vi "AnalogDemultiplexer_NI5771_3Ghz_Resonance.vi"() -> ()   [LabVIEW 2014]
uses:
  <vilib>/Platform/TimedLoop/XDataNode/timing_clust.ctl
  <vilib>/Platform/TimedLoop/XDataNode/nitl_modes.ctl
  <vilib>/Platform/TimedLoop/XDataNode/wakeup.ctl
  <vilib>/rvi/Emulation/niFpgaGetClockAttributes.vi
  <vilib>/rvi/Emulation/niFpgaSctlEmulationGetInTimedLoop.vi
  <vilib>/rvi/Emulation/niFpgaEmulationReportErrorSimple.vi
  <vilib>/rvi/eio/common/nirviEmuTemplateMethod_errors.vi
  <vilib>/rvi/Emulation/niFpgaCriticalErrorInLSC.vi
  <vilib>/rvi/Emulation/niFpgaEmulationIsFPGAContextNoSignature.vi
  <vilib>/rvi/FIFO/Fifo_Resource/nirvififoEmulationSetSize.vi
  <vilib>/rvi/DataTransferAndStorage/Container/Common/niFpgaContainerGetUniqueNameForEmu.vi
  <vilib>/rvi/FIFO/Fifo_Resource/nirviFifoEmulationQueueMgr.vi
  <instcachedir>/0/nirviFifoEmulationQueueMgr_E5CAEC123FF24DC58D834DCA3CDAA9B5.lvgen/nirviFifoEmulationQueueMgr_E5CAEC123FF24DC58D834DCA3CDAA9B5_002.vi
  <vilib>/rvi/Emulation/niFpgaProcessEmulError.vi
  <vilib>/rvi/errors/niFpgaSetErrorForExecOnDevCompSimple.vi
  <vilib>/rvi/eio/common/nirviEmuReportErrorAndStop.vi
  <vilib>/rvi/FIFO/Fifo_Resource/nirvififoEmulationCreateLock.vi
  <vilib>/rvi/FIFO/Fifo_Resource/nirvififoEmulationObtainLock.vi
  <vilib>/rvi/FIFO/Fifo_Resource/nirvififoEmulationReleaseLock.vi
  <vilib>/rvi/occurrence/nirviWaitOnOccurrenceBase.vi
  <vilib>/rvi/errors/nirviReportUnexpectedCaseInternalError.vi
  <vilib>/rvi/errors/nirviReportUnexpectedCaseInternalError (U32).vi
  <vilib>/rvi/interface/RandomDataEmulation/niFpgaRandomDataHandleErrors.vi
  <vilib>/rvi/FIFO/Fifo_Resource/nirvififoEmulationDetermineInputValidOut.vi
  <vilib>/eio/EIONode/EIONode.xnode
  <vilib>/rvi/DataTransferAndStorage/Container/XNode/niFpgaContainer.xnode
  <vilib>/rvi/FIFO/Fifo_Resource/nirvififoEmulationClear.vi
  <vilib>/Platform/TimedLoop/XDataNode/XDataNode.xnode
  <vilib>/rvi/FIFO/Fifo_Resource/nirvififoEmulationRead.vi
  <vilib>/rvi/interface/RandomDataEmulation/nirviRandomDataFpgaReadWriteTemplate.vi
  <vilib>/rvi/FIFO/Fifo_Resource/nirvififoEmulationWrite.vi
  <vilib>/Platform/TimedLoop/XDataNode/XDNodeRunTimeDep.lvlib
panel:
  in  "CutoffU8 Ch2":u8
  in  "CutoffU8 Ch1":u8
  out "ToHostA2FIFO Overflow":bool
  out "ToHostA1FIFO Overflow":bool
  out "Pixel counter A2":u32
  out "Pixel counter A1":u32
  out "InterloopFIFO Overflow":bool
  in  "BaselineU8 Ch2":u8
  in  "BaselineU8 Ch1":u8
  out "InterloopFIFO timeout":bool
  in  "Clear Interloop FIFO":bool
  out "Acquiring":bool
  in  "Wait for trigger":bool
  in  "Acquire":bool
  in  "Requested pixels A2":u32=100000 caption="Requested pixels"
  in  "Acquire continuously":bool=TRUE
  in  "Requested pixels A1":u32=100000 caption="Requested pixels"
  in  "Samples per pixel":u16=10000 caption="Samples per pixel Acq"
  out "IO Module\\AI Over Range":bool
  in  "User Command Commit":bool
  in  "User Command":u8
  out "User Command Idle":bool
  out "User Command Status":u8
  in  "User Data 0":u16
  in  "User Data 1":u8
  out "PLL Locked":bool
  out "User Error":bool
  out "Configured?":bool
  # "5771 IO module configuration"
  # "Analog demultiplexer V2"
  # "Acquisition control"
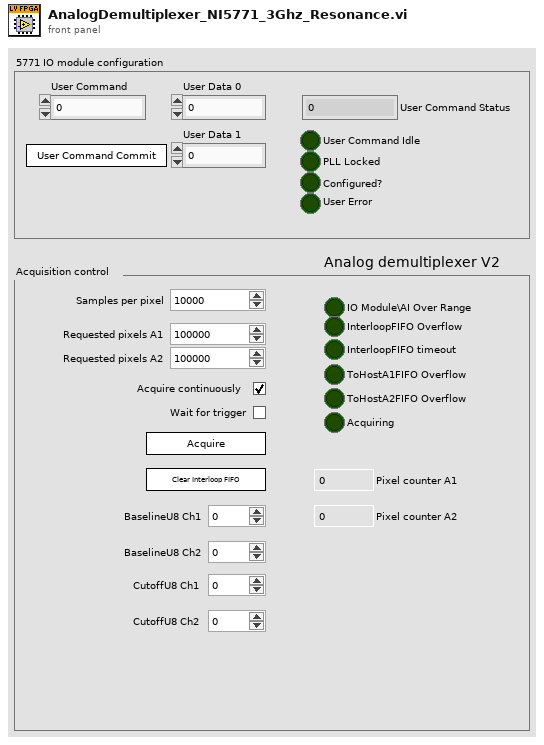
[diagram p1: front panel]
types:
  T1 = typedef "XDNodeRunTimeDep.lvlib/timing_clust.ctl" = cluster{"Expected End [f-1]":u64, "Actual End [f-1]":u64, "Finished Late? [f-1]":bool, "Expected End [i-1]":u64, "Actual End [i-1]":u64, "Finished Late? [i-1]":bool, "Expected Start [i]":u64, "Actual Start [i]":u64, "Expected Start [f]":u64, "Actual Start [f]":u64, "Source Name":string, "Structure Name":string, "Period":i64, "Deadline":i64, "Offset":i64, "Start":i64, "Priority":i32, "Timeout":i32, "Mode":T2, "Wakeup Reason":T3, "Error":errorcluster, "Source Type":string, "Secondary Source Type":string, "Global End Time":u64, "Global Start Time":u64, "Frame Duration":u64, "Iteration Duration":u64, "Assigned CPU":i32, "I/O Scan Engine Mode":u32}
  T2 = typedef "XDNodeRunTimeDep.lvlib/nitl_modes.ctl" = enum32{"No Change", "Process missed periods, maintain original phase", "Discard missed periods, maintain original phase", "Process missed periods, ignore original phase", "Discard missed periods, ignore original phase"}
  T3 = typedef "XDNodeRunTimeDep.lvlib/wakeup.ctl" = enum32{"Normal", "Aborted", "Asynchronous wakeup", "Timing source error", "Timed loop error", "Timeout"}
  T4 = cluster{"IO Module\\AI 1 Data N-7":u8, "IO Module\\AI 1 Data N-6":u8, "IO Module\\AI 1 Data N-5":u8, "IO Module\\AI 1 Data N-4":u8, "IO Module\\AI 1 Data N-3":u8, "IO Module\\AI 1 Data N-2":u8, "IO Module\\AI 1 Data N-1":u8, "IO Module\\AI 1 Data N":u8, "IO Module\\Synchronous Trigger Input":u8}
  T5 = cluster{"IO Module\\AI 0 Data N-7":u8, "IO Module\\AI 0 Data N-6":u8, "IO Module\\AI 0 Data N-5":u8, "IO Module\\AI 0 Data N-4":u8, "IO Module\\AI 0 Data N-3":u8, "IO Module\\AI 0 Data N-2":u8, "IO Module\\AI 0 Data N-1":u8, "IO Module\\AI 0 Data N":u8, "IO Module\\Synchronous Trigger Input":u8}
  T6 = cluster{u16, u16, u16, u16, u16, u16, u16, u16, "IO Module\\Synchronous Trigger Input":u8}
  T7 = cluster{"Output":u32, "Output":u32, "Output":u32, "Output":u32}
  T8 = cluster{"A1 Ch1":u32, "A1 Ch2":u32, "A2 Ch1":u32, "A2 Ch2":u32}
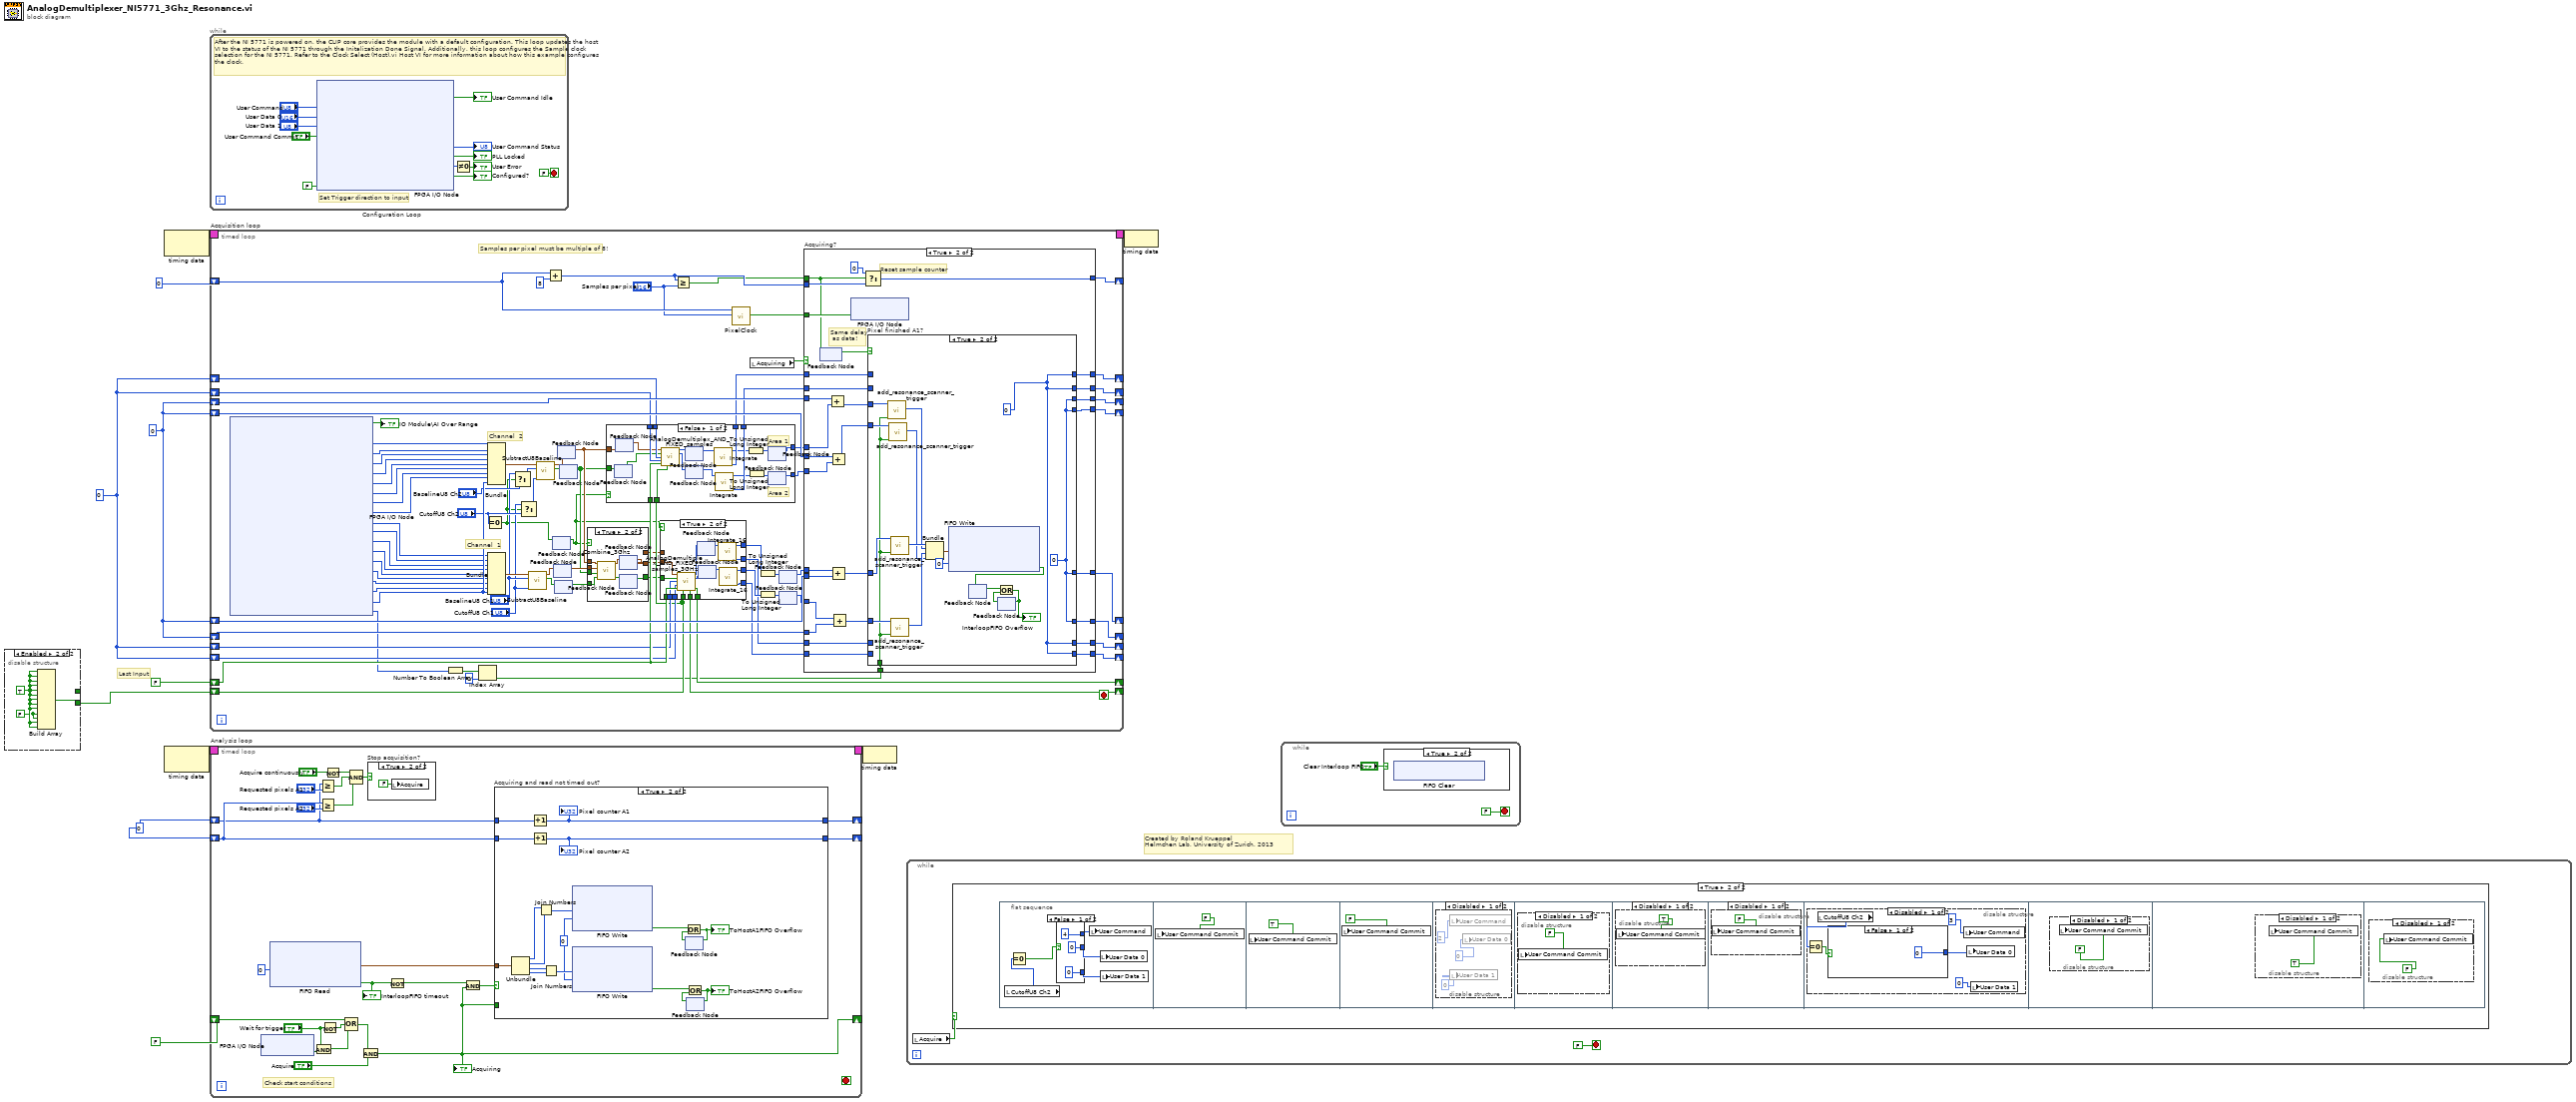
[diagram p0: block diagram]
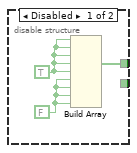
[diagram p2: hidden frame]
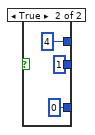
[diagram p4: hidden frame]
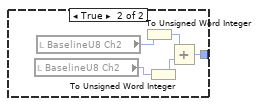
[diagram p9: hidden frame]
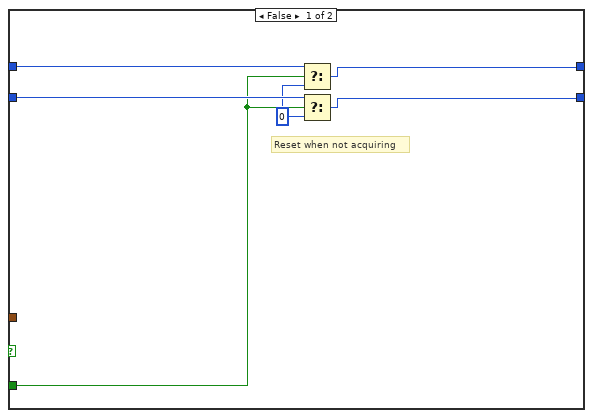
[diagram p15: hidden frame]
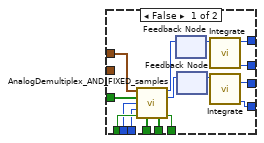
[diagram p17: hidden frame]
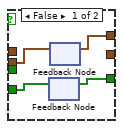
[diagram p18: hidden frame]
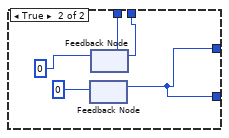
[diagram p19: hidden frame]
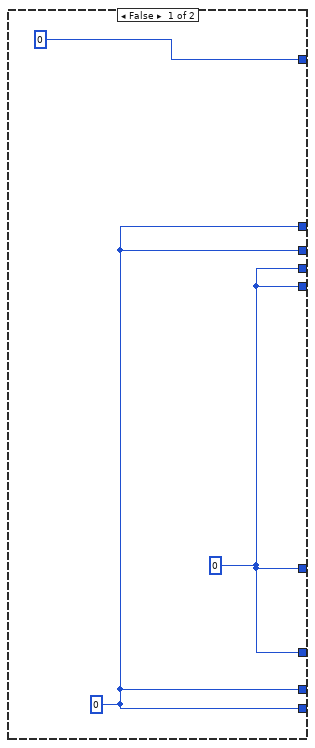
[diagram p20: hidden frame]
diagram:
  w2 = u8 0
  w4 = u32 0
  w6 = u32 0 ("Integrator out")
  # "Last Input"
  # "Created by Roland Krueppel\nHelmchen Lab, University of Zurich, 2013"
  n1 = disable-structure shown="Enabled" {
    disable-tunnel: [w14 _] -> _
    disable-tunnel: [_ w15] -> w1
    frame Disabled {
      w12 = FALSE
      w13 = TRUE
      n2 = Build Array(w13, w13, w13, w13, w13, w12, w12, w12, w12) -> (w14:bool[])
    }
    frame Enabled {
      w16 = FALSE
      w17 = TRUE
      n3 = Build Array(w17, w17, w17, w17, w17, w17, w17, w17, w17, w16, w16, w17, w17) -> (w15:bool[])
    }
  }
  n4 = node-c288() -> (w11:T1)  [unwired: 1 in]
  n5 = node-c288() -> (w9:T1)  [unwired: 1 in]
  n6 = while "Configuration Loop" {
    stop <- FALSE stop-if-true
    # "Set Trigger direction to input"
    # "After the NI 5771 is powered on, the CLIP core provides the module with a default configuration. This loop updates the host VI to the status of the NI 5771 through the Initalization Done Signal. Additionally, this loop configures the Sample clock selection for the NI 5771. Refer to the Clock Select (Host).vi Host VI for more information about how this example configures the clock."
    n7 = xnode "FPGA I/O Node"("IO Module\\User Command"="User Command", "IO Module\\User Data 0"="User Data 0", "IO Module\\User Data 1"="User Data 1", "IO Module\\User Command Commit"="User Command Commit", "IO Module\\Trigger WE"=FALSE ("IO Module\\Trigger WE")) -> ("IO Module\\User Command Idle"=→"User Command Idle":bool, "IO Module\\User Command Status"=→"User Command Status":u8, "IO Module\\PLL Locked"=→"PLL Locked":bool, "IO Module\\User Error"=w24:u8, "IO Module\\Initialization Done"=→"Configured?":bool)  [unwired: 10 in, 10 out]
    n8 = Not Equal To 0?(x=w24) -> (x != 0?=→"User Error":bool)
  }
  n9 = timed-loop "Acquisition loop" {
    timing: w11 -> [_]
    timing-out: [_] -> w10
    shift-right: [w112] -> _
    shift-left: u16 0 -> [w107]
    shift-right: [w92] -> _
    shift-left: w4 -> [w101]
    shift-right: [w91] -> _
    shift-left: w4 -> [w100]
    shift-right: [w93] -> _
    shift-left: w4 -> [w102]
    shift-right: [w94] -> _
    shift-left: w4 -> [w103]
    shift-right: [w84] -> _
    shift-left: FALSE -> [w90]
    shift-right: [w87] -> _
    shift-left: w2 -> [w78]
    shift-right: [w86] -> _
    shift-left: w2 -> [w77]
    shift-right: [w89] -> _
    shift-left: w2 -> [w79]
    shift-right: [w88] -> _
    shift-left: w2 -> [w80]
    shift-right: [w76] -> _
    shift-left: w1 -> [w75]
    stop <- _ stop-if-true
    # "Channel  2"
    # "Channel  1"
    # "Samples per pixel must be multiple of 8!"
    n10 = xnode "FPGA I/O Node"() -> ("IO Module\\AI Over Range"=→"IO Module\\AI Over Range":bool, "IO Module\\AI 1 Data N-7"=w71:u8, "IO Module\\AI 1 Data N-6"=w70:u8, "IO Module\\AI 1 Data N-5"=w69:u8, "IO Module\\AI 1 Data N-4"=w68:u8, "IO Module\\AI 1 Data N-3"=w67:u8, "IO Module\\AI 1 Data N-2"=w66:u8, "IO Module\\AI 1 Data N-1"=w65:u8, "IO Module\\AI 1 Data N"=w64:u8, "IO Module\\AI 0 Data N-7"=w62:u8, "IO Module\\AI 0 Data N-6"=w61:u8, "IO Module\\AI 0 Data N-5"=w60:u8, "IO Module\\AI 0 Data N-4"=w59:u8, "IO Module\\AI 0 Data N-3"=w58:u8, "IO Module\\AI 0 Data N-2"=w57:u8, "IO Module\\AI 0 Data N-1"=w56:u8, "IO Module\\AI 0 Data N"=w55:u8, "IO Module\\Synchronous Trigger Input"=w63:u8, "IO Module\\DIO Port 0 Rd Data"=w54:u8)  [unwired: 19 in, 19 out]
    n11 = Number To Boolean Array(number=w54) -> (Boolean array=w53:bool[])
    n12 = Index Array(array=w53, index=0) -> (element=w73:bool)
    n13 = Equal To 0?(x="CutoffU8 Ch2") -> (x = 0?=w39:bool)
    n14 = Bundle("IO Module\\AI 1 Data N-7"=w71, "IO Module\\AI 1 Data N-6"=w70, "IO Module\\AI 1 Data N-5"=w69, "IO Module\\AI 1 Data N-4"=w68, "IO Module\\AI 1 Data N-3"=w67, "IO Module\\AI 1 Data N-2"=w66, "IO Module\\AI 1 Data N-1"=w65, "IO Module\\AI 1 Data N"=w64, "IO Module\\Synchronous Trigger Input"=w63) -> (w51:T4)  [unwired: 1 in]
    n15 = Bundle("IO Module\\AI 0 Data N-7"=w62, "IO Module\\AI 0 Data N-6"=w61, "IO Module\\AI 0 Data N-5"=w60, "IO Module\\AI 0 Data N-4"=w59, "IO Module\\AI 0 Data N-3"=w58, "IO Module\\AI 0 Data N-2"=w57, "IO Module\\AI 0 Data N-1"=w56, "IO Module\\AI 0 Data N"=w55, "IO Module\\Synchronous Trigger Input"=w63) -> (w72:T5)  [unwired: 1 in]
    n16 = Select(t="BaselineU8 Ch1", s=w39, f="BaselineU8 Ch2") -> (s? t:f=w38:u8)
    n17 = Select(t="CutoffU8 Ch1", s=w39, f="CutoffU8 Ch2") -> (s? t:f=w40:u8)
    n18 = call "SubtractU8Baseline.vi"("Cutoff U8"="CutoffU8 Ch1", "Baseline U8"="BaselineU8 Ch1", "Analog data cluster in"=w72) -> ("Over? Array"=w83:bool[], "Analog data cluster out"=w108:T5)  [unwired: 7 in]
    n19 = call "SubtractU8Baseline.vi"("Cutoff U8"=w40, "Baseline U8"=w38, "Analog data cluster in"=w51) -> ("Over? Array"=w47:bool[], "Analog data cluster out"=w48:T5)  [unwired: 7 in]
    n20 = Add(x=w107, y=u16 8) -> (x+y=w110:u16)
    n21 = feedback #1() -> (w35:bool)  [unwired: 1 in]
    n22 = feedback-in #1(w39) -> ()
    n23 = feedback #2() -> (w50:T5)  [unwired: 1 in]
    n24 = feedback-in #2(w108) -> ()
    n25 = feedback #3() -> (w49:bool[])  [unwired: 1 in]
    n26 = feedback-in #3(w83) -> ()
    n27 = feedback #4() -> (w46:T5)  [unwired: 1 in]
    n28 = feedback-in #4(w48) -> ()
    n29 = feedback #5() -> (w45:bool[])  [unwired: 1 in]
    n30 = feedback-in #5(w47) -> ()
    n31 = case shown="True" w35 {
      tunnel: w50 -> [w145 w156]
      tunnel: w49 -> [w148 w155]
      tunnel: [_ w150] -> w37
      tunnel: [w147 w149] -> w36
      tunnel: w45 -> [_ w154]
      tunnel: w46 -> [_ w153]
      tunnel: [w146 _] -> w34
      frame False {
        n32 = feedback #6() -> (w147:bool[])  [unwired: 1 in]
        n33 = feedback-in #6(w148) -> ()
        n34 = feedback #7() -> (w146:T5)  [unwired: 1 in]
        n35 = feedback-in #7(w145) -> ()
      }
      frame True {
        n36 = call "Combine_3Ghz.vi"("Over? Array AI0"=w155, "Over? Array AI1"=w154, "A0 cluster in"=w156, "A1 cluster in"=w153) -> ("Over? Array Out"=w151:bool[], "A0 cluster out"=w152:T6)  [unwired: 6 in]
        n37 = feedback #8() -> (w150:T6)  [unwired: 1 in]
        n38 = feedback-in #8(w152) -> ()
        n39 = feedback #9() -> (w149:bool[])  [unwired: 1 in]
        n40 = feedback-in #9(w151) -> ()
      }
    }
    n41 = case shown="False" w35 {
      tunnel: [w176 w177] -> w98
      tunnel: [w175 w177] -> w97
      tunnel: w90 -> [w174 _]
      tunnel: [w173 w178] -> w82
      tunnel: [w172 w178] -> w81
      tunnel: w80 -> [w171 _]
      tunnel: w79 -> [w170 _]
      tunnel: w75 -> [w169 _]
      tunnel: w46 -> [w157 _]
      tunnel: w45 -> [w160 _]
      frame False {
        # "Area 2"
        # "Area 1"
        n42 = feedback #10() -> (w159:bool[])  [unwired: 1 in]
        n43 = feedback-in #10(w160) -> ()
        n44 = feedback #11() -> (w158:T5)  [unwired: 1 in]
        n45 = feedback-in #11(w157) -> ()
        n46 = call "AnalogDemultiplex_AND_FIXED_samples.vi"("Analog data cluster"=w158, "Over? Array"=w159, "Last Sample A1"=w170, "Last Sample A2"=w171, "Last? Input"=w174, "array in"=w169) -> ("Data A1 out"=w166:u64, "Data A2 out"=w164:u64)  [unwired: 6 in, 2 out]
        n47 = feedback #12() -> (w165:u64)  [unwired: 1 in]
        n48 = feedback-in #12(w166) -> ()
        n49 = feedback #13() -> (w163:u64)  [unwired: 1 in]
        n50 = feedback-in #13(w164) -> ()
        n51 = call "Integrate.vi"("New samples in"=w165) -> ("Next Sample"=w172:u8, "Sum out"=w162:u16)  [unwired: 9 in]
        n52 = call "Integrate.vi"("New samples in"=w163) -> ("Next Sample"=w173:u8, "Sum out"=w161:u16)  [unwired: 9 in]
        n53 = To Unsigned Long Integer(number=w162) -> (unsigned 32bit integer=w168:u32)
        n54 = To Unsigned Long Integer(number=w161) -> (unsigned 32bit integer=w167:u32)
        n55 = feedback #14() -> (w176:u32)  [unwired: 1 in]
        n56 = feedback-in #14(w168) -> ()
        n57 = feedback #15() -> (w175:u32)  [unwired: 1 in]
        n58 = feedback-in #15(w167) -> ()
      }
      frame True {
        n59 = feedback #16() -> (w177:u32)  [unwired: 1 in]
        n60 = feedback-in #16(u32 0) -> ()
        n61 = feedback #17() -> (w178:u8)  [unwired: 1 in]
        n62 = feedback-in #17(u8 0) -> ()
      }
    }
    n63 = case shown="True" w35 {
      tunnel: [w115 w134] -> w33
      tunnel: [w116 w133] -> w32
      tunnel: w90 -> [w128 w139]
      tunnel: [w127 w144] -> w84
      tunnel: w78 -> [w126 w138]
      tunnel: w77 -> [w125 w137]
      tunnel: [w124 w143] -> w76
      tunnel: w75 -> [w123 w142]
      tunnel: w37 -> [_ w141]
      tunnel: w36 -> [w122 w140]
      tunnel: w34 -> [w121 _]
      tunnel: [w114 w130] -> w31
      tunnel: [w113 w129] -> w30
      frame False {
        n64 = call "AnalogDemultiplex_AND_FIXED_samples.vi"("Analog data cluster"=w121, "Over? Array"=w122, "Last Sample A1"=w126, "Last Sample A2"=w125, "Last? Input"=w128, "array in"=w123) -> ("Data A1 out"=w117:u64, "Data A2 out"=w118:u64, "array out"=w124:bool[], "Last? Output"=w127:bool)  [unwired: 6 in]
        n65 = feedback #18() -> (w119:u64)  [unwired: 1 in]
        n66 = feedback-in #18(w117) -> ()
        n67 = feedback #19() -> (w120:u64)  [unwired: 1 in]
        n68 = feedback-in #19(w118) -> ()
        n69 = call "Integrate.vi"("New samples in"=w119) -> ("Next Sample"=w114:u8, "Sum out"=w115:u16)  [unwired: 9 in]
        n70 = call "Integrate.vi"("New samples in"=w120) -> ("Next Sample"=w113:u8, "Sum out"=w116:u16)  [unwired: 9 in]
      }
      frame True {
        n71 = call "AnalogDemultiplex_AND_FIXED_samples_3GHz.vi"("Analog data cluster"=w141, "Over? Array"=w140, "Last Sample A1"=w138, "Last Sample A2"=w137, "Last? Input"=w139, "array in"=w142) -> ("Data A1 out"=w136:u64, "Data A2 out"=w131:u64, "array out"=w143:bool[], "Last? Output"=w144:bool)  [unwired: 6 in]
        n72 = feedback #20() -> (w135:u64)  [unwired: 1 in]
        n73 = feedback-in #20(w136) -> ()
        n74 = feedback #21() -> (w132:u64)  [unwired: 1 in]
        n75 = feedback-in #21(w131) -> ()
        n76 = call "Integrate_16.vi"("New samples in"=w135) -> ("Next Sample"=w130:u8, "Sum out"=w134:u16)  [unwired: 9 in]
        n77 = call "Integrate_16.vi"("New samples in"=w132) -> ("Next Sample"=w129:u8, "Sum out"=w133:u16)  [unwired: 9 in]
      }
    }
    n78 = Greater Or Equal?(x=w110, y="Samples per pixel") -> (x >= y?=w109:bool)
    n79 = call "PixelClock.vi"("Samples per pixel"="Samples per pixel", "Sample counter"=w107) -> ("Pixel clock"=w106:bool)  [unwired: 9 in]
    n80 = local read "Acquiring"() -> (w95:bool)
    n81 = To Unsigned Long Integer(number=w33) -> (unsigned 32bit integer=w105:u32)
    n82 = To Unsigned Long Integer(number=w32) -> (unsigned 32bit integer=w104:u32)
    n83 = feedback #22() -> (w99:u32)  [unwired: 1 in]
    n84 = feedback-in #22(w105) -> ()
    n85 = feedback #23() -> (w96:u32)  [unwired: 1 in]
    n86 = feedback-in #23(w104) -> ()
    n87 = case "Acquiring?" shown="True" w95 {
      tunnel: [u16 0 ("t") w214] -> w112
      tunnel: w110 -> [_ w213]
      tunnel: w109 -> [_ w203]
      tunnel: w106 -> [_ w207]
      tunnel: w103 -> [_ w193]
      tunnel: w102 -> [_ w212]
      tunnel: w101 -> [_ w196]
      tunnel: w100 -> [_ w211]
      tunnel: w99 -> [_ w194]
      tunnel: w98 -> [_ w210]
      tunnel: w97 -> [_ w209]
      tunnel: w96 -> [_ w195]
      tunnel: [w183 w201] -> w94
      tunnel: [w183 w200] -> w93
      tunnel: [w183 w199] -> w92
      tunnel: [w183 w198] -> w91
      tunnel: [w181 w192] -> w89
      tunnel: [w181 w191] -> w88
      tunnel: [w181 w190] -> w87
      tunnel: [w181 w189] -> w86
      tunnel: w81 -> [_ w188]
      tunnel: w82 -> [_ w187]
      tunnel: w30 -> [_ w186]
      tunnel: w31 -> [_ w185]
      tunnel: w73 -> [_ w184]
      frame False {
        w181 = u8 0 ("t")
        w183 = u32 0
      }
      frame True {
        # "Same delay\n as data!"
        # "Reset sample counter"
        n88 = feedback #24() -> (w202:bool)  [unwired: 1 in]
        n89 = feedback-in #24(w203) -> ()
        n90 = Add(x=w212, y=w210) -> (x+y=w205:u32)
        n91 = Add(x=w211, y=w209) -> (x+y=w204:u32)
        n92 = Add(x=w194, y=w193) -> (x+y=w206:u32)
        n93 = Add(x=w195, y=w196) -> (x+y=w197:u32)
        n94 = xnode "FPGA I/O Node"("Pixel clock"=w207) -> ()  [unwired: 1 in, 1 out]
        n95 = Select(t=u16 0, s=w203, f=w213) -> (s? t:f=w214:u16)
        n96 = case "Pixel finished A1?" shown="True" w202 {
          tunnel: w206 -> [w222 w231]
          tunnel: w205 -> [w221 w229]
          tunnel: w197 -> [w220 w233]
          tunnel: w204 -> [w219 w227]
          tunnel: [w222 w234] -> w201
          tunnel: [w221 w234] -> w200
          tunnel: [w220 w234] -> w199
          tunnel: [w219 w234] -> w198
          tunnel: [w218 w223] -> w192
          tunnel: [w217 w223] -> w191
          tunnel: [w215 w223] -> w190
          tunnel: [w216 w223] -> w189
          tunnel: w188 -> [w218 _]
          tunnel: w187 -> [w217 _]
          tunnel: w186 -> [w216 _]
          tunnel: w185 -> [w215 _]
          tunnel: w184 -> [_ w225]
          frame False {
          }
          frame True {
            w223 = u8 0
            w234 = u32 0
            n97 = call "add_resonance_scanner_trigger.vi"("Trigger"=w225, "Input"=w229) -> ("Output"=w228:u32)  [unwired: 9 in]
            n98 = call "add_resonance_scanner_trigger.vi"("Trigger"=w225, "Input"=w227) -> ("Output"=w226:u32)  [unwired: 9 in]
            n99 = call "add_resonance_scanner_trigger.vi"("Trigger"=w225, "Input"=w231) -> ("Output"=w230:u32)  [unwired: 9 in]
            n100 = call "add_resonance_scanner_trigger.vi"("Trigger"=w225, "Input"=w233) -> ("Output"=w232:u32)  [unwired: 9 in]
            n101 = Bundle("Output"=w230, "Output"=w228, "Output"=w232, "Output"=w226) -> (w224:T7)  [unwired: 1 in]
            n102 = xnode ("FIFO Write")("Element"=w224, "Timeout"=0) -> ("Timed Out?"=w235:bool)  [unwired: 1 in, 1 out]
            n103 = feedback #25() -> (w236:bool)  [unwired: 1 in]
            n104 = feedback-in #25(w235) -> ()
            n105 = feedback #26() -> (w237:bool)  [unwired: 1 in]
            n106 = Or(x=w236, y=w237) -> (x .or. y?=w238:bool)
            "InterloopFIFO Overflow" <- w238
            n107 = feedback-in #26(w238) -> ()
          }
        }
      }
    }
  }
  n108 = timed-loop "Analysis loop" {
    timing: w9 -> [_]
    timing-out: [_] -> w8
    shift-right: [w242] -> _
    shift-left: FALSE -> [w252]
    shift-right: [w245] -> _
    shift-left: w6 -> [w246]
    shift-right: [w244] -> _
    shift-left: w6 -> [w247]
    stop <- _ stop-if-true
    # "Check start conditions"
    n109 = xnode "FPGA I/O Node"() -> ("TriggerIn"=w257:bool)  [unwired: 1 in, 1 out]
    n110 = xnode ("FIFO Read")("Timeout"=0) -> ("Element"=w243:T8, "Timed Out?"=w249:bool)  [unwired: 1 in, 1 out]
    "InterloopFIFO timeout" <- w249
    n111 = And(x="Wait for trigger", y=w257) -> (x .and. y?=w254:bool)
    n112 = Greater Or Equal?(x=w246, y="Requested pixels A1") -> (x >= y?=w260:bool)
    n113 = Greater Or Equal?(x=w247, y="Requested pixels A2") -> (x >= y?=w259:bool)
    n114 = Not(x="Wait for trigger") -> (.not. x?=w255:bool)
    n115 = Not(x="Acquire continuously") -> (.not. x?=w261:bool)
    n116 = Compound Arithmetic op=OR(w252, w255, w254) -> (w253:bool)
    n117 = Compound Arithmetic op=AND(w261, w260, w259) -> (w251:bool)
    n118 = And(x=w253, y="Acquire") -> (x .and. y?=w242:bool)
    "Acquiring" <- w242
    n119 = case "Stop acquisition?" shown="True" w251 {
      frame False {
      }
      frame True {
        n120 = local write "Acquire"(FALSE ("Acquire")) -> ()
      }
    }
    n121 = Not(x=w249) -> (.not. x?=w248:bool)
    n122 = And(x=w248, y=w242) -> (x .and. y?=w250:bool)
    n123 = case "Acquiring and read not timed out?" shown="True" w250 {
      tunnel: w247 -> [w269 w288]
      tunnel: w246 -> [w271 w289]
      tunnel: [w270 w286] -> w245
      tunnel: [w268 w287] -> w244
      tunnel: w243 -> [_ w285]
      tunnel: w242 -> [w267 _]
      frame False {
        w266 = u32 0 ("f")
        # "Reset when not acquiring"
        n124 = Select(t=w271, s=w267, f=w266) -> (s? t:f=w270:u32)
        n125 = Select(t=w269, s=w267, f=w266) -> (s? t:f=w268:u32)
      }
      frame True {
        w278 = 0 ("Timeout")
        n126 = Unbundle(w285) -> ("A1 Ch1"=w284:u32, "A1 Ch2"=w283:u32, "A2 Ch1"=w281:u32, "A2 Ch2"=w280:u32)
        n127 = Increment(x=w289) -> (x+1=w286:u32)
        "Pixel counter A1" <- w286
        n128 = Increment(x=w288) -> (x+1=w287:u32)
        "Pixel counter A2" <- w287
        n129 = Join Numbers(hi=w284, lo=w283) -> ((hi.lo)=w282:u64)
        n130 = Join Numbers(hi=w281, lo=w280) -> ((hi.lo)=w279:u64)
        n131 = xnode ("FIFO Write")("Element"=w282, "Timeout"=w278) -> ("Timed Out?"=w276:bool)  [unwired: 1 in, 1 out]
        n132 = xnode ("FIFO Write")("Element"=w279, "Timeout"=w278) -> ("Timed Out?"=w272:bool)  [unwired: 1 in, 1 out]
        n133 = feedback #27() -> (w275:bool)  [unwired: 1 in]
        n134 = Or(x=w276, y=w275) -> (x .or. y?=w277:bool)
        "ToHostA1FIFO Overflow" <- w277
        n135 = feedback-in #27(w277) -> ()
        n136 = feedback #28() -> (w273:bool)  [unwired: 1 in]
        n137 = Or(x=w272, y=w273) -> (x .or. y?=w274:bool)
        "ToHostA2FIFO Overflow" <- w274
        n138 = feedback-in #28(w274) -> ()
      }
    }
  }
  n139 = node-c288(w8) -> ()
  n140 = while {
    stop <- FALSE stop-if-true
    n141 = local read "Acquire"() -> (w293:bool)
    n142 = case shown="True" w293 {
      frame False {
      }
      frame True {
        n143 = flat-sequence {
          frame #0 {
            n144 = local read "CutoffU8 Ch2"() -> (w296:u8)
            n145 = Equal To 0?(x=w296) -> (x = 0?=w295:bool)
            n146 = case shown="False" w295 {
              tunnel: [u8 0 u8 0] -> w299
              tunnel: [u16 0 u16 1] -> w298
              tunnel: [u8 4 u8 4] -> w297
              frame False {
              }
              frame True {
              }
            }
            n147 = local write "User Command"(w297) -> ()
            n148 = local write "User Data 0"(w298) -> ()
            n149 = local write "User Data 1"(w299) -> ()
          }
          frame #1 {
            n150 = local write "User Command Commit"(FALSE) -> ()
          }
          frame #2 {
            n151 = local write "User Command Commit"(TRUE) -> ()
          }
          frame #3 {
            n152 = local write "User Command Commit"(FALSE) -> ()
          }
          frame #4 {
            n153 = disable-structure shown="Disabled" {
              frame Disabled {
                n154 = local write "User Command"(u8 2) -> ()
                n155 = local write "User Data 1"(u8 0) -> ()
                n156 = local write "User Data 0"(u8 0) -> ()
              }
              frame Enabled {
              }
            }
          }
          frame #5 {
            n157 = disable-structure shown="Disabled" {
              frame Disabled {
                n158 = local write "User Command Commit"(FALSE) -> ()
              }
              frame Enabled {
              }
            }
          }
          frame #6 {
            n159 = disable-structure shown="Disabled" {
              frame Disabled {
                n160 = local write "User Command Commit"(TRUE) -> ()
              }
              frame Enabled {
              }
            }
          }
          frame #7 {
            n161 = disable-structure shown="Disabled" {
              frame Disabled {
                n162 = local write "User Command Commit"(FALSE) -> ()
              }
              frame Enabled {
              }
            }
          }
          frame #8 {
            n163 = disable-structure shown="Disabled" {
              frame Disabled {
                n164 = local read "CutoffU8 Ch2"() -> (w316:u8)
                n165 = Equal To 0?(x=w316) -> (x = 0?=w315:bool)
                n166 = case shown="False" w315 {
                  tunnel: [u16 0 w325] -> w319
                  frame False {
                  }
                  frame True {
                    n167 = local read "BaselineU8 Ch2"() -> (w324:u8)
                    n168 = local read "BaselineU8 Ch2"() -> (w321:u8)
                    n169 = To Unsigned Word Integer(number=w321) -> (unsigned 16bit integer=w322:u16)
                    n170 = To Unsigned Word Integer(number=w324) -> (unsigned 16bit integer=w323:u16)
                    n171 = Add(x=w322, y=w323) -> (x+y=w325:u16)
                  }
                }
                n172 = local write "User Command"(u8 3) -> ()
                n173 = local write "User Data 0"(w319) -> ()
                n174 = local write "User Data 1"(u8 0) -> ()
              }
              frame Enabled {
              }
            }
          }
          frame #9 {
            n175 = disable-structure shown="Disabled" {
              frame Disabled {
                n176 = local write "User Command Commit"(FALSE) -> ()
              }
              frame Enabled {
              }
            }
          }
          frame #10 {
            n177 = disable-structure shown="Disabled" {
              frame Disabled {
                n178 = local write "User Command Commit"(TRUE) -> ()
              }
              frame Enabled {
              }
            }
          }
          frame #11 {
            n179 = disable-structure shown="Disabled" {
              frame Disabled {
                n180 = local write "User Command Commit"(FALSE) -> ()
              }
              frame Enabled {
              }
            }
          }
        }
      }
    }
  }
  n181 = node-c288(w10) -> ()
  n182 = while {
    stop <- FALSE stop-if-true
    n183 = case shown="True" "Clear Interloop FIFO" {
      frame False {
      }
      frame True {
        n184 = xnode ("FIFO Clear")() -> ()  [unwired: 1 in, 1 out]
      }
    }
  }
